vi "VisitOxideSites.vi"(0 "Microsites":T2(array[cluster]), 4 "Path":path, 7 "UiDefinition":T1, 13 "CurrentPositionIndex":i32) -> (10 "IV":dbl[][](array[numeric]))   [LabVIEW 2020]
uses:
  UIReferences.ctl
  C:/Users/User/Desktop/Automation/NextVersion4/LabviewDXFViewer/bin/Release/LabviewDXFViewer.exe
  LabviewDXFViewer/bin/Release/LabviewDXFViewer.exe
  <vilib>/Utility/file.llb/Write Delimited Spreadsheet (string).vi
  <vilib>/Utility/file.llb/Write Delimited Spreadsheet (DBL).vi
panel:
  out "error out":errorcluster
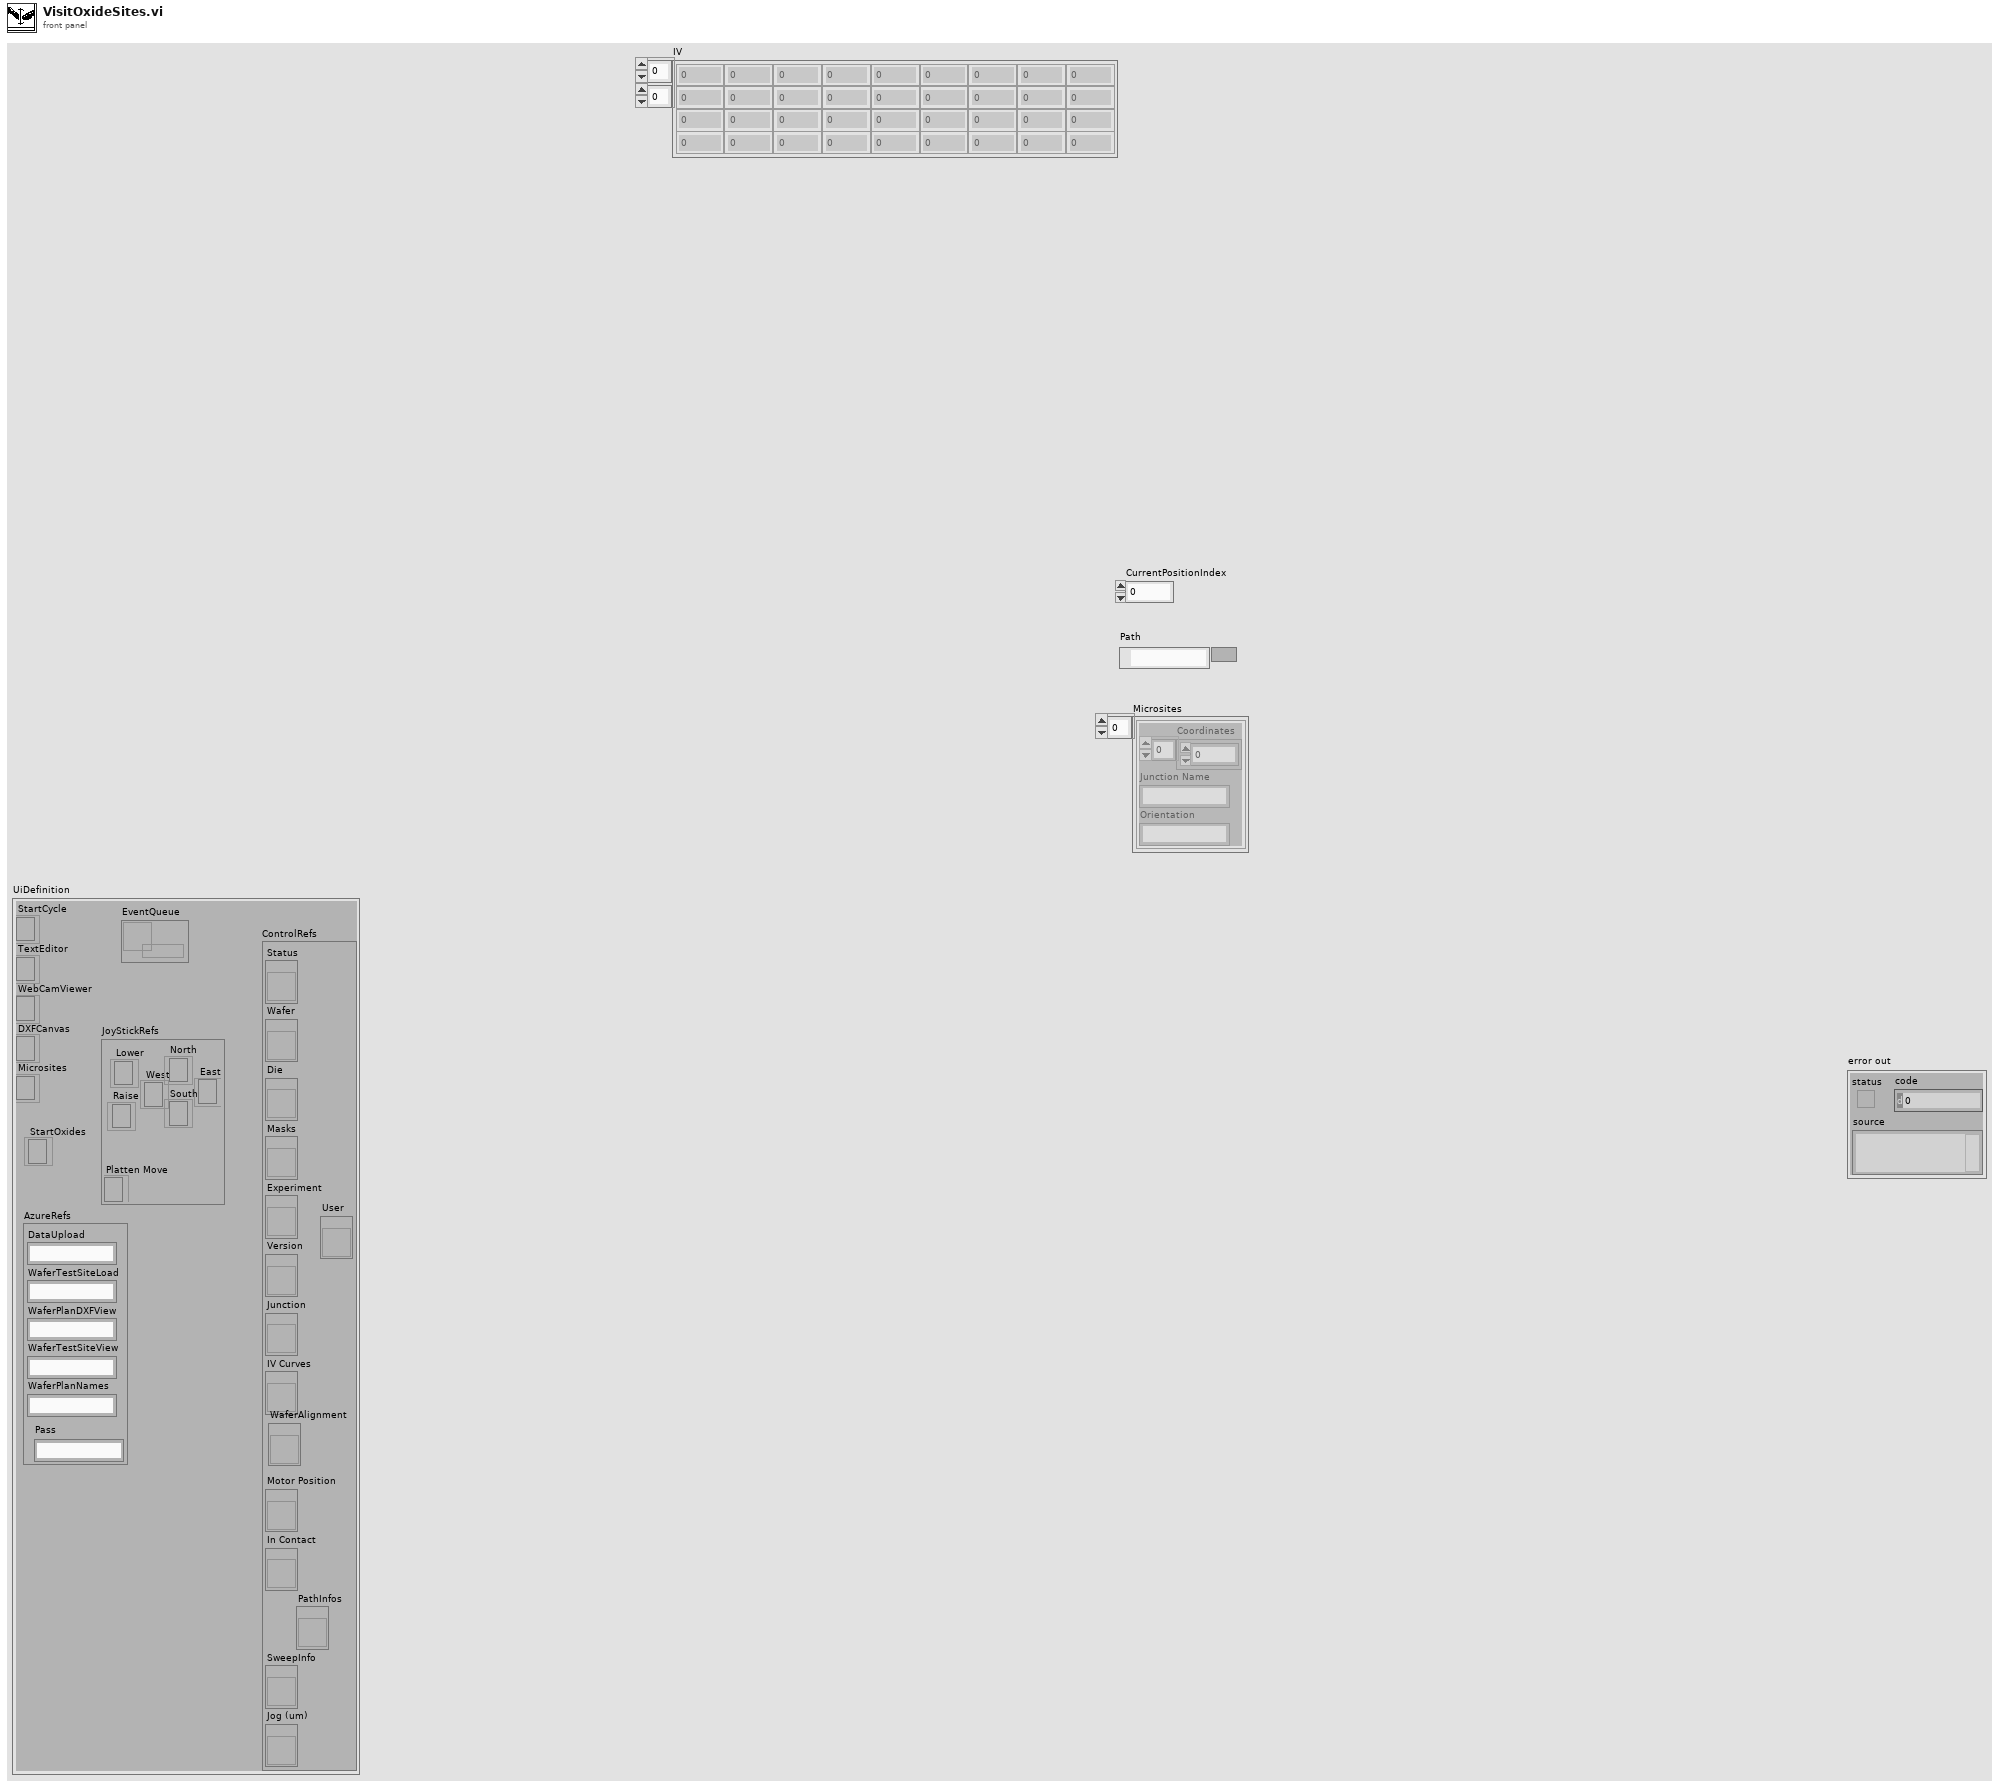
[diagram p1: front panel]
types:
  T1 = typedef "UIReferences.ctl" = cluster{"StartCycle":refnum<k24>, "TextEditor":refnum<k24>, "WebCamViewer":refnum<k24>, "DXFCanvas":refnum<k24>, "Microsites":refnum<k24>, "JoyStickRefs":cluster{"North":refnum<k24>, "Lower":refnum<k24>, "Raise":refnum<k24>, "Platten Move":refnum<k24>, "West":refnum<k24>, "East":refnum<k24>, "South":refnum<k24>}, "AzureRefs":cluster{"DataUpload":string, "WaferTestSiteLoad":string, "WaferPlanDXFView":string, "WaferTestSiteView":string, "WaferPlanNames":string, "Pass":string}, "ControlRefs":cluster{"Status":refnum<vi>, "Wafer":refnum<vi>, "Die":refnum<vi>, "Masks":refnum<vi>, "Experiment":refnum<vi>, "Version":refnum<vi>, "Junction":refnum<vi>, "IV Curves":refnum<vi>, "Motor Position":refnum<vi>, "In Contact":refnum<vi>, "SweepInfo":refnum<vi>, "Jog (um)":refnum<vi>, "PathInfos":refnum<vi>, "User":refnum<vi>, "WaferAlignment":refnum<vi>}, "EventQueue":refnum<queue>, "StartOxides":refnum<k24>}
  T2 = cluster{"Coordinates":dbl[], "Junction Name":string, "Orientation":string}[]
  T3 = cluster{"Coordinates":dbl[], "Junction Name":string, "Orientation":string}
  T4 = typedef "WaferAlignmentType.ctl" = cluster{"Wafer Units to microns":dbl, "Rotation Misalign":dbl[], "Scale Misalign":dbl, "Steps Per micron":dbl, "Position 1":i32[], "Chip Orientation":i32, "Position 2":i32[], "Lift Distance":i32, "Position 3":i32[], "Jog Height":i32}
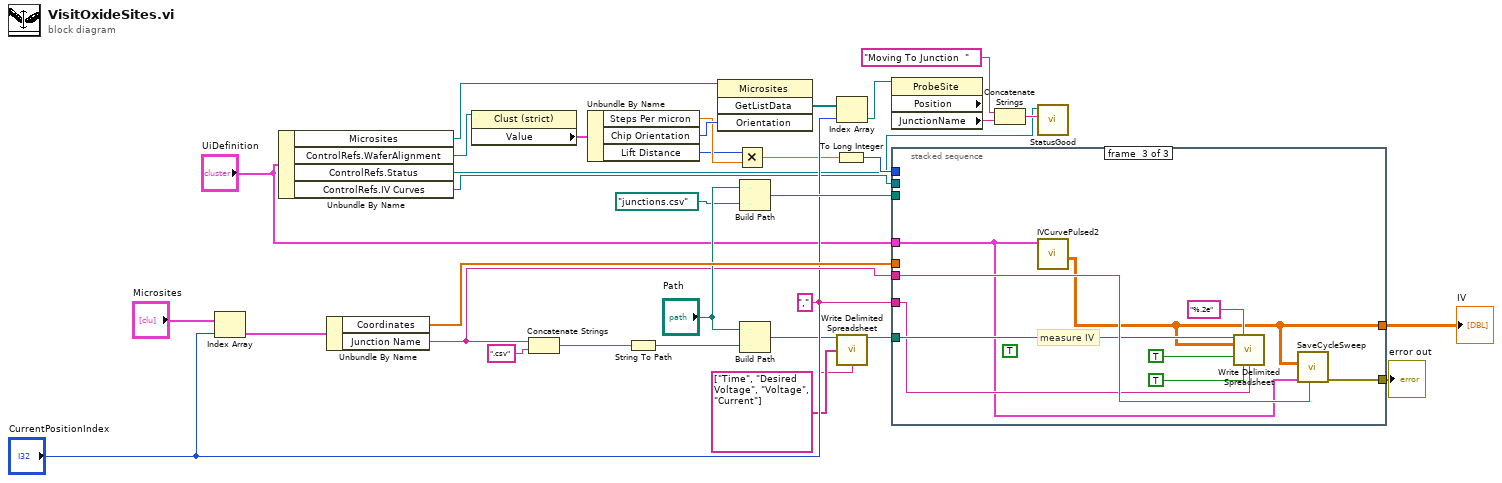
[diagram p0: block diagram]
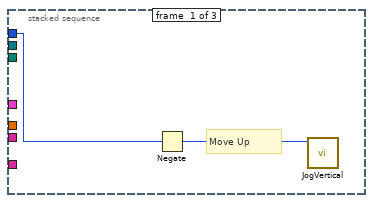
[diagram p2: hidden frame]
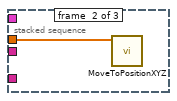
[diagram p3: hidden frame]
diagram:
  w4 = "," ("delimiter (\\t)")
  n1 = Index Array(array="Microsites", index="CurrentPositionIndex") -> (element=w23:T3)
  n2 = Unbundle By Name("UiDefinition") -> ("Microsites"=w3:refnum<k24>, "ControlRefs.WaferAlignment"=w17:refnum<vi>, "ControlRefs.Status"=w14:refnum<vi>, "ControlRefs.IV Curves"=w10:refnum<vi>)
  n3 = Unbundle By Name(w23) -> ("Coordinates"=w31:dbl[], "Junction Name"=w25:string)
  n4 = property class="Clust (strict)"(reference=w17) -> ("Value"=w16:T4)  [unwired: 1 in, 2 out]
  n5 = Concatenate Strings(w25, ".csv" ("string")) -> (w30:string)
  n6 = Unbundle By Name(w16) -> ("Steps Per micron"=w12:dbl, "Chip Orientation"=w15:i32, "Lift Distance"=w11:i32)
  n7 = String To Path(string=w30) -> (path=w29:path)
  n8 = invoke class="Microsites" method="GetListData"(reference=w3, "Orientation"=w15) -> ("GetListData"=w18:refnum<k24>[])  [unwired: 2 in, 3 out]
  n9 = Multiply(x=w11, y=w12) -> (x*y=w13:dbl)
  n10 = Build Path(base path="Path", name or relative path=path "junctions.csv") -> (appended path=w32:path)
  n11 = Build Path(base path="Path", name or relative path=w29) -> (appended path=w7:path)
  n12 = To Long Integer(number=w13) -> (32bit integer=w33:i32)
  n13 = Index Array(array=w18, index="CurrentPositionIndex") -> (element=w2:refnum<k24>)
  n14 = call-poly <vilib>:"Write Delimited Spreadsheet.vi"("file path (dialog if empty)"=w7, "1D data"=string[] ["Time", "Desired Voltage", "Voltage", "Current"], "delimiter (\\t)"=w4) -> ("new file path (Not A Path if cancelled)"=w5:path)  [unwired: 11 in, 1 out]
  n15 = property class="ProbeSite" props=["Position", "JunctionName"](reference=w2) -> ("JunctionName"=w22:string)  [unwired: 1 in, 3 out]
  n16 = stacked-sequence {
    tunnel: w33 -> [w34 _ _]
    tunnel: w32 -> [_ _ _]
    tunnel: w31 -> [_ w36 _]
    tunnel: w25 -> [_ _ w45]
    tunnel: w5 -> [_ _ w44]
    tunnel: w10 -> [_ _ _]
    tunnel: "UiDefinition" -> [_ _ w38]
    tunnel: [_ _ w41] -> w8
    tunnel: w4 -> [_ _ w39]
    tunnel: [_ _ w37] -> w1
    frame #0 {
      # "Move Up"
      n17 = Negate(x=w34) -> (-x=w35:i32)
      n18 = call "JogVertical.vi"("Numeric"=w35) -> ()  [unwired: 11 in]
    }
    frame #1 {
      n19 = call "MoveToPositionXYZ.vi"("Array"=w36) -> ()  [unwired: 11 in]
    }
    frame #2 {
      (unwired) TRUE ("Reprogram")
      # "measure IV"
      n20 = call "IVCurvePulsed2.vi"("UiDefinition"=w38) -> ("appended array"=w37:dbl[][])  [unwired: 9 in, 1 out]
      n21 = call-poly <vilib>:"Write Delimited Spreadsheet.vi"("file path (dialog if empty)"=w44, "format (%.3f)"="%.2e", "2D data"=w37, "append to file? (new file:F)"=TRUE, "transpose? (no:F)"=TRUE, "delimiter (\\t)"=w39) -> ()  [unwired: 8 in, 2 out]
      n22 = call "SaveCycleSweep.vi"("JunctionName"=w45, "UiDefinition 2"=w38, "appended array"=w37) -> ("error out"=w41:errorcluster)  [unwired: 8 in]
    }
  }
  "error out" <- w8
  "IV" <- w1
  n23 = Concatenate Strings("Moving To Junction  " ("Text.Text"), w22) -> (w21:string)
  n24 = call "StatusGood.vi"("Text.Text"=w21, "String in"=w14) -> ()  [unwired: 10 in]
